vi "SUM 1.vi"() -> ()   [LabVIEW 2011]
panel:
  out "0404A0ER":u8=150 format="%.0x"
  out "0404A0EQ":u8=147 format="%.0x"
  out "0404A0EP":u8=144 format="%.0x"
  out "0404A0EN":u8=142 format="%.0x"
  out "0404A0EM":u8=203 format="%.0x"
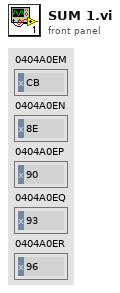
[diagram p1: front panel]
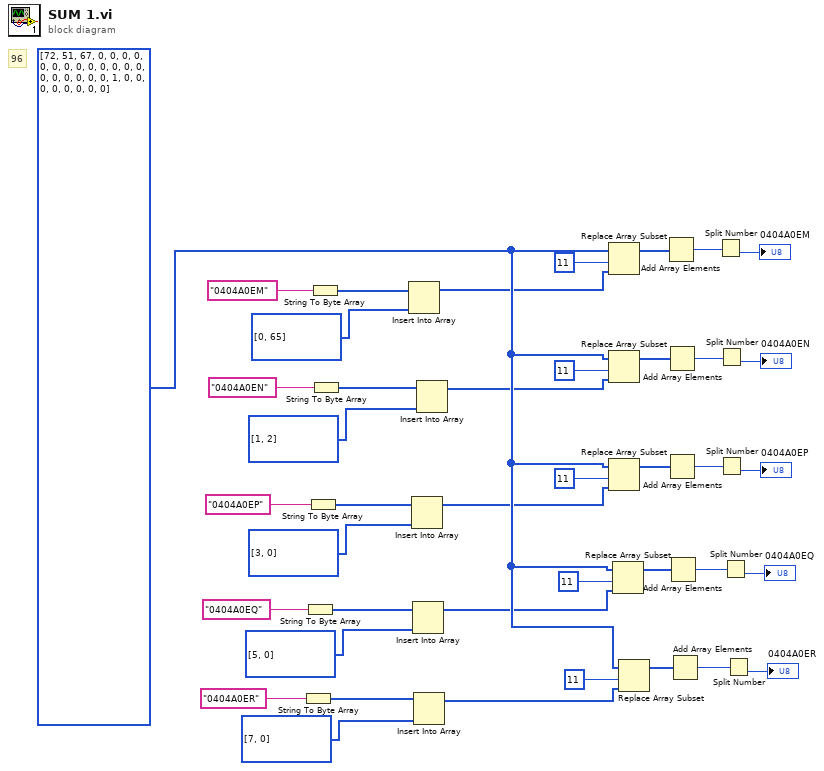
[diagram p0: block diagram]
diagram:
  w31 = u8[] [72, 51, 67, 0, 0, 0, 0, 0, 0, 0, 0, 0, 0, 0, 0, 0, 0, 0, 0, 0, 0, 0, 1, 0, 0, 0, 0, 0, 0, 0, 0] ("数组")
  # "107"
  # "126"
  # "125"
  # "120"
  # "115"
  # "116"
  # "111"
  # "110"
  # "106"
  # "105"
  # "98"
  # "101"
  # "100"
  # "96"
  n1 = String To Byte Array(string="0404A0ER") -> (unsigned byte array=w18:u8[])
  n2 = String To Byte Array(string="0404A0EQ") -> (unsigned byte array=w21:u8[])
  n3 = String To Byte Array(string="0404A0EP") -> (unsigned byte array=w24:u8[])
  n4 = String To Byte Array(string="0404A0EM") -> (unsigned byte array=w30:u8[])
  n5 = String To Byte Array(string="0404A0EN") -> (unsigned byte array=w27:u8[])
  n6 = Insert Into Array(array=w30, new element=u8[] [0, 65] ("数组")) -> (w28:u8[])  [unwired: 1 in]
  n7 = Insert Into Array(array=w24, new element=u8[] [3, 0] ("数组")) -> (w22:u8[])  [unwired: 1 in]
  n8 = Insert Into Array(array=w21, new element=u8[] [5, 0] ("数组")) -> (w20:u8[])  [unwired: 1 in]
  n9 = Insert Into Array(array=w18, new element=u8[] [7, 0] ("数组")) -> (w17:u8[])  [unwired: 1 in]
  n10 = Insert Into Array(array=w27, new element=u8[] [1, 2] ("数组")) -> (w25:u8[])  [unwired: 1 in]
  n11 = Replace Array Subset(array=w31, new element=w28, index=11) -> (w15:u8[])
  n12 = Replace Array Subset(array=w31, new element=w25, index=11) -> (w14:u8[])
  n13 = Replace Array Subset(array=w31, new element=w22, index=11) -> (w13:u8[])
  n14 = Replace Array Subset(array=w31, new element=w20, index=11) -> (w12:u8[])
  n15 = Replace Array Subset(array=w31, new element=w17, index=11) -> (w11:u8[])
  n16 = Add Array Elements(numeric array=w15) -> (sum=w10:u8)
  n17 = Add Array Elements(numeric array=w14) -> (sum=w7:u8)
  n18 = Add Array Elements(numeric array=w13) -> (sum=w5:u8)
  n19 = Add Array Elements(numeric array=w12) -> (sum=w3:u8)
  n20 = Add Array Elements(numeric array=w11) -> (sum=w1:u8)
  n21 = Split Number(x=w10) -> (lo(x)=→"0404A0EM":u8)  [unwired: 1 out]
  n22 = Split Number(x=w7) -> (lo(x)=→"0404A0EN":u8)  [unwired: 1 out]
  n23 = Split Number(x=w5) -> (lo(x)=→"0404A0EP":u8)  [unwired: 1 out]
  n24 = Split Number(x=w3) -> (lo(x)=→"0404A0EQ":u8)  [unwired: 1 out]
  n25 = Split Number(x=w1) -> (lo(x)=→"0404A0ER":u8)  [unwired: 1 out]
